vi "GetClosestFullscreenDisplayMode.vi"(4 "Include High Density Modes":bool caption="Include High Density Modes (F)", 6 "Refresh Rate":sgl caption="Refresh Rate (0.0: Desktop Refresh Rate)", 8 "No Error":errorcluster, 9 "h":i32, 10 "w":i32, 11 "DisplayID":T2) -> (0 "Error Out":errorcluster, 3 "Closest Full Screen Display Mode":T1)   [LabVIEW 2026, in "SDL3.lvlib" / "Video.lvlib"]
doc: "<B>Summary</B>\nGet the closest match to the requested display mode.\n\n<B>Remarks</B>\nThe available display modes are scanned and closest is filled in with the closest mode matching the requested mode and returned. The mode format and refresh rate default to the desktop mode if they are set to 0. The modes are scanned with size being first priority, format being second priority, and finally checking the refresh rate. If all the available modes are too small, then false is returned."
uses:
  Video.lvlib
  DisplayID--integer.ctl
  DisplayMode--cluster.ctl
  Pixels/PixelFormat--enum.ctl
  f2a002a6-6479-4e1d-9d36-2d0676373c84.vi
  74da5f93-18bf-4d33-b977-ba1e4be2821d.vi
  Pixels/U32ToPixelFormatEnum.vi
  <vilib>/Utility/error.llb/Error Cluster From Error Code.vi
  Error/Error.lvlib
  Lib/SDL3.dll
  Pixels/Pixels.lvlib
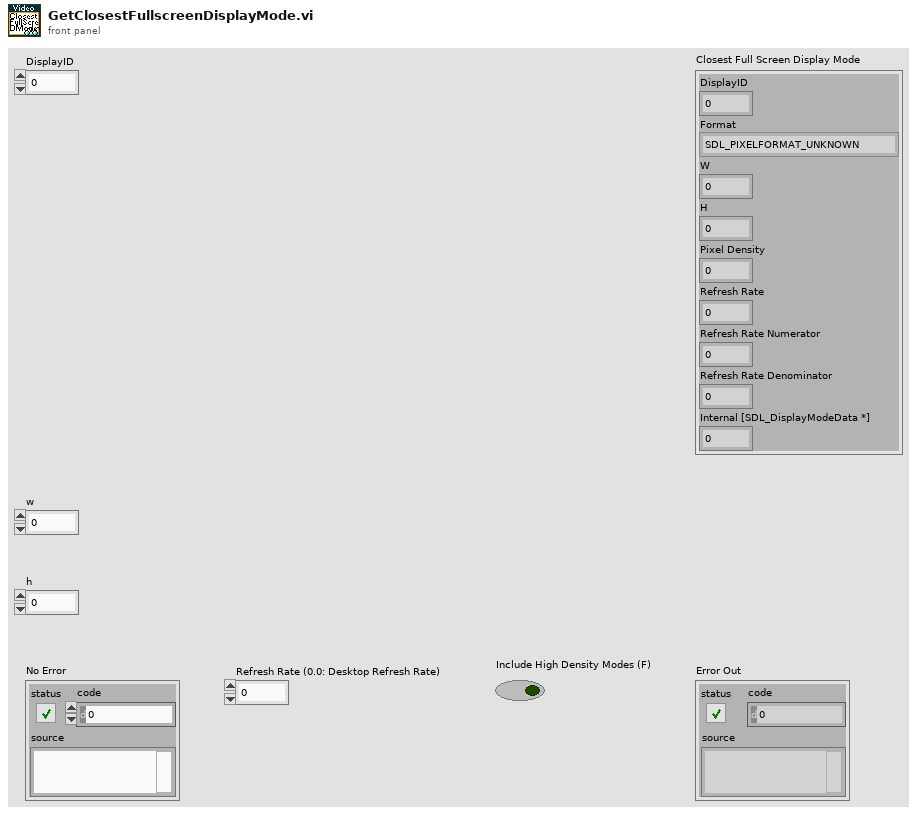
[diagram p1: front panel]
types:
  T1 = typedef "SDL3.lvlib/Video.lvlib/DisplayMode--cluster.ctl" = cluster{"DisplayID":T2, "Format":T3, "W":i32, "H":i32, "Pixel Density":sgl, "Refresh Rate":sgl, "Refresh Rate Numerator":i32, "Refresh Rate Denominator":i32, "Internal [SDL_DisplayModeData *]":i64}
  T2 = typedef "SDL3.lvlib/Video.lvlib/DisplayID--integer.ctl" = u32
  T3 = typedef "SDL3.lvlib/Pixels.lvlib/PixelFormat--enum.ctl" = enum32{"SDL_PIXELFORMAT_UNKNOWN", "SDL_PIXELFORMAT_INDEX1LSB", "SDL_PIXELFORMAT_INDEX1MSB", "SDL_PIXELFORMAT_INDEX2LSB", "SDL_PIXELFORMAT_INDEX2MSB", "SDL_PIXELFORMAT_INDEX4LSB", "SDL_PIXELFORMAT_INDEX4MSB", "SDL_PIXELFORMAT_INDEX8", "SDL_PIXELFORMAT_RGB332", "SDL_PIXELFORMAT_XRGB4444", "SDL_PIXELFORMAT_XBGR4444", "SDL_PIXELFORMAT_XRGB1555", "SDL_PIXELFORMAT_XBGR1555", "SDL_PIXELFORMAT_ARGB4444", "SDL_PIXELFORMAT_RGBA4444", "SDL_PIXELFORMAT_ABGR4444", "SDL_PIXELFORMAT_BGRA4444", "SDL_PIXELFORMAT_ARGB1555", "SDL_PIXELFORMAT_RGBA5551", "SDL_PIXELFORMAT_ABGR1555", "SDL_PIXELFORMAT_BGRA5551", "SDL_PIXELFORMAT_RGB565", "SDL_PIXELFORMAT_BGR565", "SDL_PIXELFORMAT_RGB24", "SDL_PIXELFORMAT_BGR24", "SDL_PIXELFORMAT_XRGB8888", "SDL_PIXELFORMAT_RGBX8888", "SDL_PIXELFORMAT_XBGR8888", "SDL_PIXELFORMAT_BGRX8888", "SDL_PIXELFORMAT_ARGB8888", "SDL_PIXELFORMAT_RGBA8888", "SDL_PIXELFORMAT_ABGR8888", "SDL_PIXELFORMAT_BGRA8888", "SDL_PIXELFORMAT_XRGB2101010", "SDL_PIXELFORMAT_XBGR2101010", "SDL_PIXELFORMAT_ARGB2101010", "SDL_PIXELFORMAT_ABGR2101010", "SDL_PIXELFORMAT_RGB48", "SDL_PIXELFORMAT_BGR48", "SDL_PIXELFORMAT_RGBA64", "SDL_PIXELFORMAT_ARGB64", "SDL_PIXELFORMAT_BGRA64", "SDL_PIXELFORMAT_ABGR64", "SDL_PIXELFORMAT_RGB48_FLOAT", "SDL_PIXELFORMAT_BGR48_FLOAT", "SDL_PIXELFORMAT_RGBA64_FLOAT", "SDL_PIXELFORMAT_ARGB64_FLOAT", "SDL_PIXELFORMAT_BGRA64_FLOAT", "SDL_PIXELFORMAT_ABGR64_FLOAT", "SDL_PIXELFORMAT_RGB96_FLOAT", "SDL_PIXELFORMAT_BGR96_FLOAT", "SDL_PIXELFORMAT_RGBA128_FLOAT", "SDL_PIXELFORMAT_ARGB128_FLOAT", "SDL_PIXELFORMAT_BGRA128_FLOAT", "SDL_PIXELFORMAT_ABGR128_FLOAT", "SDL_PIXELFORMAT_YV12", "SDL_PIXELFORMAT_IYUV", "SDL_PIXELFORMAT_YUY2", "SDL_PIXELFORMAT_UYVY", "SDL_PIXELFORMAT_YVYU", "SDL_PIXELFORMAT_NV12", "SDL_PIXELFORMAT_NV21", "SDL_PIXELFORMAT_P010", "SDL_PIXELFORMAT_EXTERNAL_OES"}
  T4 = typedef "SDL3.lvlib/Video.lvlib/DisplayMode-Internal-Win32--cluster.ctl" = cluster{"DisplayID":T2, "Format":u32, "W":i32, "H":i32, "Pixel Density":sgl, "Refresh Rate":sgl, "Refresh Rate Numerator":i32, "Refresh Rate Denominator":i32, "Internal [SDL_DisplayModeData *]":i32}
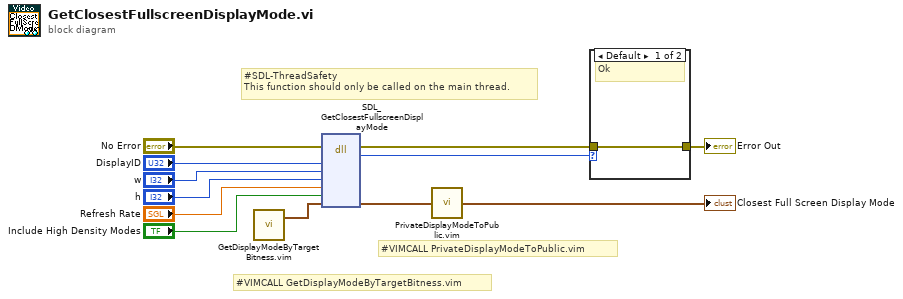
[diagram p0: block diagram]
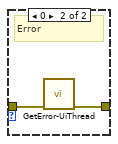
[diagram p2: hidden frame]
diagram:
  # "#VIMCALL PrivateDisplayModeToPublic.vim"
  # "#VIMCALL GetDisplayModeByTargetBitness.vim"
  # "#SDL-ThreadSafety\nThis function should only be called on the main thread."
  n1 = call "GetDisplayModeByTargetBitness.vim"() -> ("Display Mode"=w3:T4)  [unwired: 1 out]
  n2 = dll-call lib="C:/Users/saukko/Dev/LV-SDL3/Sources/SDL3/Lib/SDL3.*" fn="SDL_GetClosestFullscreenDisplayMode"(error in="No Error", "displayID"="DisplayID", "w"="w", "h"="h", "refresh_rate"="Refresh Rate", "include_high_density_modes"="Include High Density Modes", "closest"=w3) -> (error out=w10:errorcluster, "return type"=w8:i32, "closest"=w2:T4)  [unwired: 7 in, 1 out]
  n3 = call "PrivateDisplayModeToPublic.vim"("Private Display Mode"=w2) -> ("Public Display Mode"=→"Closest Full Screen Display Mode":T1)
  n4 = case shown="Default" w8 {
    tunnel: w10 -> [w13 w15]
    tunnel: [w13 w14] -> w9
    frame Default {
      # "Ok"
    }
    frame 0 {
      # "Error"
      n5 = call "GetError-UiThread.vi"("No Error"=w15) -> ("error out"=w14:errorcluster)  [unwired: 10 in]
    }
  }
  "Error Out" <- w9
